vi "Triggering Encoder.vi"(7 "Channel (1|2)":T2 items=["ENC1"=1, "ENC2"=2], 8 "error in (no error)":errorcluster, 9 "condition":T1, 10 "position":i32, 11 "MicroDAQ.lvlib:Analog Input.lvclass":refnum<class "Analog Input.lvclass">) -> (0 "error out":errorcluster, 3 "MicroDAQ.lvlib:Analog Input.lvclass out":refnum<class "Analog Input.lvclass">)   [LabVIEW 2009, in "MicroDAQ.lvlib" / "Analog Input.lvclass"]
doc: "This function configures Encoder value trigger for AO/AI scan operation. The module argument determines which encoder module position value will be used. The slope argument defines if trigger shall occur for value greater or lower then position argument."
uses:
  <instrlib>/MicroDAQ/Channel/Analog Input/Analog Input.lvclass
  <instrlib>/MicroDAQ/Tools/Encoder type.ctl
  <instrlib>/MicroDAQ/Tools/Trigger Encoder condition enum.ctl
  <instrlib>/MicroDAQ/Tools/Trigger type.ctl
  <instrlib>/MicroDAQ/Channel/Channel.lvclass
  <instrlib>/MicroDAQ/Mlink library wraper/mlink.lvlib
  <instrlib>/MicroDAQ/MicroDAQ.lvlib
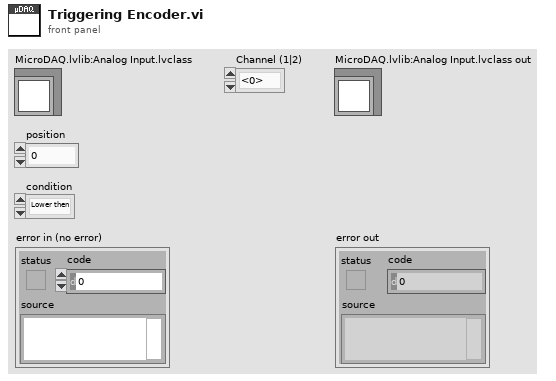
[diagram p1: front panel]
types:
  T1 = typedef "MicroDAQ.lvlib/Trigger Encoder condition enum.ctl" = enum16{"Lower then", "Greater then"}
  T2 = typedef "MicroDAQ.lvlib/Encoder type.ctl" = u8
  T3 = typedef "MicroDAQ.lvlib/Trigger type.ctl" = enum8{"Analog output", "Analog input"}
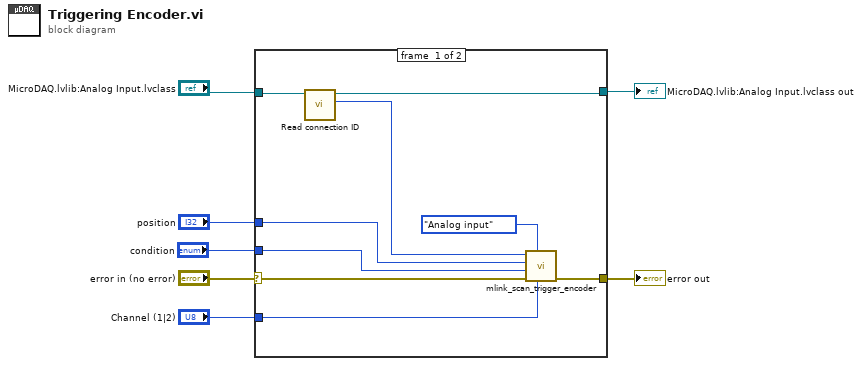
[diagram p0: block diagram]
diagram:
  n1 = case shown="No Error" "error in (no error)" {
    selector: "error in (no error)" -> [w14 w17]
    tunnel: [w13 w17] -> w6
    tunnel: [w15 w18] -> w5
    tunnel: "MicroDAQ.lvlib:Analog Input.lvclass" -> [w16 w18]
    tunnel: "Channel (1|2)" -> [w10 _]
    tunnel: "position" -> [w9 _]
    tunnel: "condition" -> [w8 _]
    frame #0 {
      n2 = call <instrlib>:"Read connection ID.vi"("Task in"=w16) -> ("connection ID"=w11:i32, "Task out"=w15:refnum<class "Analog Input.lvclass">)  [unwired: 9 in]
      n3 = call <instrlib>:"mlink_scan_trigger_encoder.vi"("module"=w10, "trigger type"=Trigger_type."Analog input", "error in (no error)"=w14, "slope"=w8, "position"=w9, "connection ID"=w11) -> ("error out"=w13:errorcluster)  [unwired: 4 in, 1 out]
    }
    frame #1 {
    }
  }
  "error out" <- w6
  "MicroDAQ.lvlib:Analog Input.lvclass out" <- w5
